vi "Begin.vi"(8 "error in":errorcluster) -> (0 "error out":errorcluster)   [LabVIEW 2018]
doc: "Called before other user functions, this VI is expected to open initial I/O refnums, load in file data, and do all program initialization. Notice that the <B>error out</B> terminal is simply used for data flow. Wiring it to other structures or subVIs ensures that this VI runs first."
uses:
  <vilib>/Rock Robotics/WPI/ThirdParty/Phoenix-LabVIEW/Motor Controller/Controls/CTRE_Phoenix_MotorControl_EnhancedMotorControllerConfigurables.ctl
  <vilib>/Rock Robotics/WPI/ThirdParty/Phoenix-LabVIEW/Motor Controller/Controls/CTRE_Phoenix_MotorControl_BaseConfigurables.ctl
  <vilib>/Rock Robotics/WPI/ThirdParty/Phoenix-LabVIEW/Motor Controller/Controls/CTRE_Phoenix_MotorControl_VelocityMeasurementPeriod.ctl
  <vilib>/Rock Robotics/WPI/ThirdParty/Phoenix-LabVIEW/Motor Controller/Controls/CTRE_Phoenix_MotorControl_SlotStructure.ctl
  <vilib>/Rock Robotics/WPI/ThirdParty/Phoenix-LabVIEW/Motor Controller/Controls/CTRE_Phoenix_MotorControl_FilterStruct.ctl
  <vilib>/Rock Robotics/WPI/ThirdParty/Phoenix-LabVIEW/Motor Controller/Controls/CTRE_Phoenix_MotorControl_RemoteSourceType.ctl
  <vilib>/Rock Robotics/WPI/ThirdParty/Phoenix-LabVIEW/Controls/CTRE_Phoenix_CustomParamConfiguration.ctl
  <vilib>/Rock Robotics/WPI/ThirdParty/Phoenix-LabVIEW/Motor Controller/Controls/CTRE_Phoenix_MotorControl_FeedbackDevice.ctl
  <vilib>/Rock Robotics/WPI/ThirdParty/Phoenix-LabVIEW/Motor Controller/Controls/CTRE_Phoenix_MotorControl_SensorTermFeedbackDevice_Enhanced.ctl
  <vilib>/Rock Robotics/WPI/ThirdParty/Phoenix-LabVIEW/Motor Controller/Controls/CTRE_Phoenix_MotorControl_LimitSwitchNormal.ctl
  <vilib>/Rock Robotics/WPI/ThirdParty/Phoenix-LabVIEW/Motor Controller/Controls/CTRE_Phoenix_MotorControl_LimitSwitchSource_Local.ctl
  <vilib>/Rock Robotics/WPI/ThirdParty/Phoenix-LabVIEW/Motor Controller/Controls/CTRE_Phoenix_MotorControl_MotorControllerConfigurables.ctl
  <vilib>/Rock Robotics/WPI/ThirdParty/Phoenix-LabVIEW/Motor Controller/Controls/CTRE_Phoenix_MotorControl_RemoteFeedbackDevice.ctl
  <vilib>/Rock Robotics/WPI/ThirdParty/Phoenix-LabVIEW/Motor Controller/Controls/CTRE_Phoenix_MotorControl_SensorTermFeedbackDevice.ctl
  <vilib>/Rock Robotics/WPI/ThirdParty/Phoenix-LabVIEW/Motor Controller/Controls/CTRE_Phoenix_MotorControl_LimitSwitchSource.ctl
  <vilib>/Rock Robotics/WPI/DriverStation/WPI_DriverStationRobotMode2.ctl
  <vilib>/Rock Robotics/WPI/Joystick/WPI_JoystickDeviceEnum.ctl
  <vilib>/Rock Robotics/WPI/Solenoid/WPI_SolenoidChannel.ctl
  <vilib>/Rock Robotics/SystemInterfaces/AI/FPGA_AIChannel.ctl
  <vilib>/Rock Robotics/WPI/ThirdParty/Phoenix-LabVIEW/Motor Controller/Controls/CTRE_Phoenix_MotorControl_NeutralMode.ctl
  <vilib>/Rock Robotics/WPI/SafetyOutput/WPI_SafetyOutputConfigMenu.ctl
  Robot Global Data.vi
  RefNums_DriverStation.vi
  <vilib>/Rock Robotics/Network Tables/NT Write String Array.vi
  <vilib>/Rock Robotics/WPI/Solenoid/WPI_SolenoidOpenDouble.vi
  RefNums_Actuators.vi
  <vilib>/Rock Robotics/WPI/Utilities/WPI_GetSetVariantRefNum.vi
  RefNums_Sensors.vi
  <vilib>/Rock Robotics/WPI/Solenoid/WPI_SolenoidOpenSingle.vi
  <vilib>/Rock Robotics/WPI/RobotDrive/WPI_RobotDriveOpen2MotorWithExistingMotors.vi
panel:
  in  "Victor Enhanced Control":T1={"Base Configurables"={"openLoopRamp"=0.0, "closedLoopRamp"=0.0, "peakOutputForward"=1.0, "peakOutputReverse"=-1.0, "nominalOutputForward"=0.0, "nominalOutputReverse"=0.0, "neutralDeadband"=0.04, "voltageCompSaturation"=0.0, "voltageMeasurementFilter"=32, "velocityMeasurementPeriod"=100, "velocityMeasurementWindow"=64, "forwardSoftLimitThreshold"=0, "reverseSoftLimitThreshold"=0, "forwardSoftLimitEnable"=FALSE, "reverseSoftLimitEnable"=FALSE, "slot0"={"P"=0.0, "I"=0.0, "D"=0.0, "F"=0.0, "integralZone"=0.0, "allowableClosedLoopError"=0, "maxIntegralAccumulator"=0.0, "closedLoopPeakOutput"=1.0, "closedLoopPeriod"=1}, "slot1"={"P"=0.0, "I"=0.0, "D"=0.0, "F"=0.0, "integralZone"=0.0, "allowableClosedLoopError"=0, "maxIntegralAccumulator"=0.0, "closedLoopPeakOutput"=1.0, "closedLoopPeriod"=1}, "slot2"={"P"=0.0, "I"=0.0, "D"=0.0, "F"=0.0, "integralZone"=0.0, "allowableClosedLoopError"=0, "maxIntegralAccumulator"=0.0, "closedLoopPeakOutput"=1.0, "closedLoopPeriod"=1}, "slot3"={"P"=0.0, "I"=0.0, "D"=0.0, "F"=0.0, "integralZone"=0.0, "allowableClosedLoopError"=0, "maxIntegralAccumulator"=0.0, "closedLoopPeakOutput"=1.0, "closedLoopPeriod"=1}, "auxPIDPolarity"=FALSE, "remoteFilter0"={"remoteSensorDeviceID"=0, "remoteSensorSource"=enum."Off"}, "remoteFilter1"={"remoteSensorDeviceID"=0, "remoteSensorSource"=enum."Off"}, "motionCruiseVelocity"=0, "motionAcceleration"=0, "motionProfileTrajectoryPeriod"=0, "feedbackNotContinuous"=FALSE, "remoteSensorClosedLoopDisableNeutralOnLOS"=FALSE, "clearPositionOnLimitF"=FALSE, "clearPositionOnLimitR"=FALSE, "clearPositionOnQuadIdx"=FALSE, "limitSwitchDisableNeutralOnLOS"=FALSE, "softLimitDisableNeutralOnLOS"=FALSE, "pulseWidthPeriod_EdgesPerRot"=1, "pulseWidthPeriod_FilterWindowSz"=1, "customParam"={"customParam0"=0, "customParam1"=0}, "trajectoryInterpolationEnable"=TRUE}, "primaryPID"={"selectedFeedbackCoefficient"=1.0, "selectedFeedbackSensor"=11}, "auxiliaryPID"={"selectedFeedbackCoefficient"=1.0, "selectedFeedbackSensor"=11}, "sum 0 term"=11, "sum 1 term"=11, "diff 0 term "=11, "diff 1 term"=11, "forwardLimitSwitchDeviceID"=0, "reverseLimitSwitchDeviceID"=0, "forwardLimitSwitchNormal"=enum."Normally Open", "reverseLimitSwitchNormal"=enum."Normally Open", "forwardLimitSwitchSource"=3, "reverseLimitSwitchSource"=3} {"diff 1 term" items=["Remote Source 0"=11, "Remote Source 1"=12, "Software Emulated"=15]; "diff 0 term" items=["Remote Source 0"=11, "Remote Source 1"=12, "Software Emulated"=15]; "sum 1 term" items=["Remote Source 0"=11, "Remote Source 1"=12, "Software Emulated"=15]; "sum 0 term" items=["Remote Source 0"=11, "Remote Source 1"=12, "Software Emulated"=15]; "reverseLimitSwitchSource" items=["Remote Talon SRX"=1, "Remote CANifier"=2, "Deactivated"=3]; "forwardLimitSwitchSource" items=["Remote Talon SRX"=1, "Remote CANifier"=2, "Deactivated"=3]; "auxiliaryPID"."selectedFeedbackSensor" items=["Sensor Sum (S0 + S1)"=9, "Sensor Difference (D0 - D1)"=10, "Remote Source 0"=11, "Remote Source 1"=12, "Software Emulated"=15]; "primaryPID"."selectedFeedbackSensor" items=["Sensor Sum (S0 + S1)"=9, "Sensor Difference (D0 - D1)"=10, "Remote Source 0"=11, "Remote Source 1"=12, "Software Emulated"=15]; "Base Configurables"."velocityMeasurementPeriod" items=["Period_1ms"=1, "Period_2ms"=2, "Period_5ms"=5, "Period_10ms"=10, "Period_20ms"=20, "Period_25ms"=25, "Period_50ms"=50, "Period_100ms"=100]}
  in  "Talon Enhanced Config":T12={"Base Configurables"={"openLoopRamp"=0.0, "closedLoopRamp"=0.0, "peakOutputForward"=1.0, "peakOutputReverse"=-1.0, "nominalOutputForward"=0.0, "nominalOutputReverse"=0.0, "neutralDeadband"=0.04, "voltageCompSaturation"=0.0, "voltageMeasurementFilter"=32, "velocityMeasurementPeriod"=100, "velocityMeasurementWindow"=64, "forwardSoftLimitThreshold"=0, "reverseSoftLimitThreshold"=0, "forwardSoftLimitEnable"=FALSE, "reverseSoftLimitEnable"=FALSE, "slot0"={"P"=0.0, "I"=0.0, "D"=0.0, "F"=0.0, "integralZone"=0.0, "allowableClosedLoopError"=0, "maxIntegralAccumulator"=0.0, "closedLoopPeakOutput"=1.0, "closedLoopPeriod"=1}, "slot1"={"P"=0.0, "I"=0.0, "D"=0.0, "F"=0.0, "integralZone"=0.0, "allowableClosedLoopError"=0, "maxIntegralAccumulator"=0.0, "closedLoopPeakOutput"=1.0, "closedLoopPeriod"=1}, "slot2"={"P"=0.0, "I"=0.0, "D"=0.0, "F"=0.0, "integralZone"=0.0, "allowableClosedLoopError"=0, "maxIntegralAccumulator"=0.0, "closedLoopPeakOutput"=1.0, "closedLoopPeriod"=1}, "slot3"={"P"=0.0, "I"=0.0, "D"=0.0, "F"=0.0, "integralZone"=0.0, "allowableClosedLoopError"=0, "maxIntegralAccumulator"=0.0, "closedLoopPeakOutput"=1.0, "closedLoopPeriod"=1}, "auxPIDPolarity"=FALSE, "remoteFilter0"={"remoteSensorDeviceID"=0, "remoteSensorSource"=enum."Off"}, "remoteFilter1"={"remoteSensorDeviceID"=0, "remoteSensorSource"=enum."Off"}, "motionCruiseVelocity"=0, "motionAcceleration"=0, "motionProfileTrajectoryPeriod"=0, "feedbackNotContinuous"=FALSE, "remoteSensorClosedLoopDisableNeutralOnLOS"=FALSE, "clearPositionOnLimitF"=FALSE, "clearPositionOnLimitR"=FALSE, "clearPositionOnQuadIdx"=FALSE, "limitSwitchDisableNeutralOnLOS"=FALSE, "softLimitDisableNeutralOnLOS"=FALSE, "pulseWidthPeriod_EdgesPerRot"=1, "pulseWidthPeriod_FilterWindowSz"=1, "customParam"={"customParam0"=0, "customParam1"=0}, "trajectoryInterpolationEnable"=TRUE}, "primaryPID"={"selectedFeedbackCoefficient"=1.0, "selectedFeedbackSensor"=0}, "auxiliaryPID"={"selectedFeedbackCoefficient"=1.0, "selectedFeedbackSensor"=0}, "sum0Term"=0, "sum1Term"=0, "diff0Term"=0, "diff1Term"=0, "forwardLimitSwitchNormal"=enum."Normally Open", "reverseLimitSwitchNormal"=enum."Normally Open", "forwardLimitSwitchDeviceID"=0, "reverseLimitSwitchDeviceID"=0, "forwardLimitSwitchSource"=enum."Feedback Connector", "reverseLimitSwitchSource"=enum."Feedback Connector", "peakCurrentLimit"=1, "peakCurrentDuration"=1, "continuousCurrentLimit"=1} {"diff1Term" items=["QuadEncoder"=0, "Analog"=2, "Tachometer"=4, "Pulse Width Encoded Position"=8, "Remote Source 0"=11, "Remote Source 1"=12, "Software Emulated"=15]; "diff0Term" items=["QuadEncoder"=0, "Analog"=2, "Tachometer"=4, "Pulse Width Encoded Position"=8, "Remote Source 0"=11, "Remote Source 1"=12, "Software Emulated"=15]; "sum1Term" items=["QuadEncoder"=0, "Analog"=2, "Tachometer"=4, "Pulse Width Encoded Position"=8, "Remote Source 0"=11, "Remote Source 1"=12, "Software Emulated"=15]; "sum0Term" items=["QuadEncoder"=0, "Analog"=2, "Tachometer"=4, "Pulse Width Encoded Position"=8, "Remote Source 0"=11, "Remote Source 1"=12, "Software Emulated"=15]; "auxiliaryPID"."selectedFeedbackSensor" items=["QuadEncoder"=0, "Analog"=2, "Tachometer"=4, "Pulse Width Encoded Position"=8, "Sensor Sum (S0 + S1)"=9, "Sensor Difference (D0 - D1)"=10, "Remote Source 0"=11, "Remote Source 1"=12, "Software Emulated"=15]; "primaryPID"."selectedFeedbackSensor" items=["QuadEncoder"=0, "Analog"=2, "Tachometer"=4, "Pulse Width Encoded Position"=8, "Sensor Sum (S0 + S1)"=9, "Sensor Difference (D0 - D1)"=10, "Remote Source 0"=11, "Remote Source 1"=12, "Software Emulated"=15]; "Base Configurables"."velocityMeasurementPeriod" items=["Period_1ms"=1, "Period_2ms"=2, "Period_5ms"=5, "Period_10ms"=10, "Period_20ms"=20, "Period_25ms"=25, "Period_50ms"=50, "Period_100ms"=100]}
  # "Sum and Diff terms are ways to select more than one sensor as a feedback device. \n Sum 0 is the first feedback device to be used for the Sum term, \n Sum 1 is the feedback device to be added to Sum 0 for the Sum term\n Diff 0 and Diff 1 work in a similar manner"
  # "These are only applicable\nif using a remote limit switch.\n\nLocal limit switches/no limit\nswitches do not use this"
  # "False: Primary Output = PID[0] + PID[1]  ---  Auxiliary Output = PID[0] - PID[1]\nTrue:  Primary Output = PID[0] - PID[1] --- Auxiliary Output = PID[0] + PID[1]"
  # "Enable the motion profile executor to perform linear interpolation between profile points.  Defaults to True."
  # "Sum and Diff terms are ways to select more than one sensor as a feedback device. \n Sum 0 is the first feedback device to be used for the Sum term.\n Sum 1 is the feedback device to be added to Sum 0 for the Sum term.\n Diff 0 and Diff 1 work in a similar manner."
  # "These are only applicable\nif using a remote limit switch.\n\nLocal limit switches/no limit\nswitches do not use this."
  # "Current is below Continuous threshold AND\n\n(Requested output is weaker** than applied motor\noutput OR is in the opposite direction).\n/\nMotor output is set to requested output."
  # "Current is above Peak* Threshold for Peak Duration.\n/\nReduce motor output (towards neutral)."
  # "Current is below Continuous threshold.\n/\nRamp motor output towards requested output."
  # "Current is above Continuous threshold.\n/\nReduce motor output (towards neutral)."
  # "Current Limiting is NOT enabled\nby default.\nCall this VI to enable."
  # "*If the configured Peak Threshold is less than the Continuous Threshold, the applied Peak Threshold is set equal to the Configured Continuous Threshold in firmware.\n** Both requested output and applied motor output are in the same direction, and requested output is closer to neutral."
  # "False: Primary Output = PID[0] + PID[1]  ---  Auxiliary Output = PID[0] - PID[1]\nTrue:  Primary Output = PID[0] - PID[1] --- Auxiliary Output = PID[0] + PID[1]"
  # "Enable the motion profile executor to perform linear interpolation between profile points.  Defaults to True."
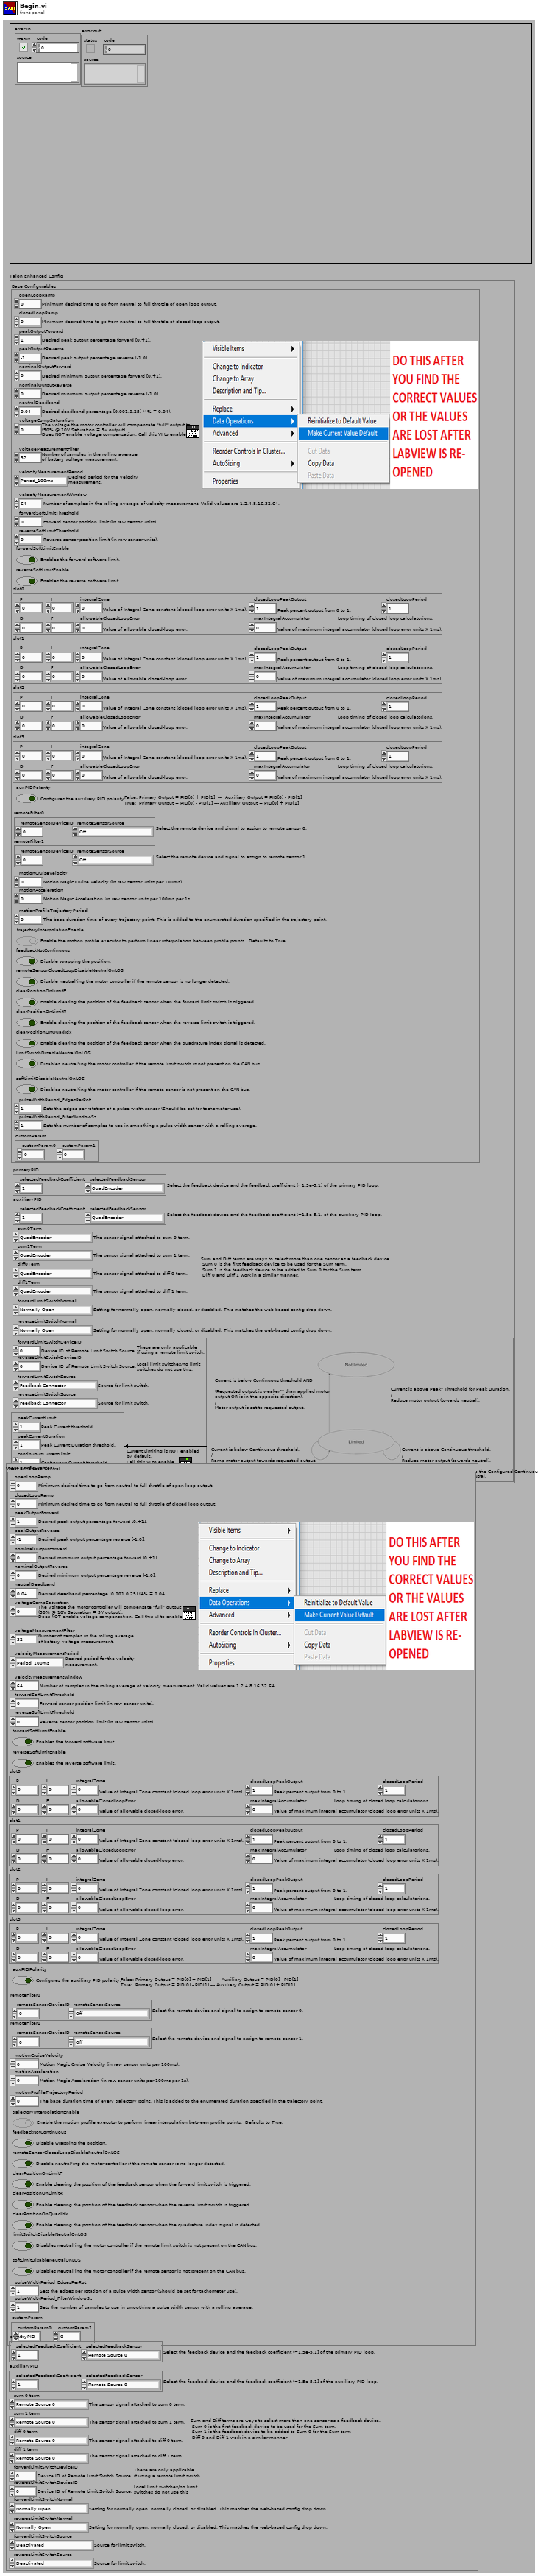
[diagram p1: front panel]
types:
  T1 = typedef "CTRE_Phoenix_MotorControl_MotorControllerConfigurables.ctl" = cluster{"Base Configurables":T2, "primaryPID":cluster{"selectedFeedbackCoefficient":dbl, "selectedFeedbackSensor":T8}, "auxiliaryPID":cluster{"selectedFeedbackCoefficient":dbl, "selectedFeedbackSensor":T8}, "sum 0 term":T9, "sum 1 term":T9, "diff 0 term ":T9, "diff 1 term":T9, "forwardLimitSwitchDeviceID":i32, "reverseLimitSwitchDeviceID":i32, "forwardLimitSwitchNormal":T10, "reverseLimitSwitchNormal":T10, "forwardLimitSwitchSource":T11, "reverseLimitSwitchSource":T11}
  T2 = typedef "CTRE_Phoenix_MotorControl_BaseConfigurables.ctl" = cluster{"openLoopRamp":dbl, "closedLoopRamp":dbl, "peakOutputForward":dbl, "peakOutputReverse":dbl, "nominalOutputForward":dbl, "nominalOutputReverse":dbl, "neutralDeadband":dbl, "voltageCompSaturation":dbl, "voltageMeasurementFilter":i32, "velocityMeasurementPeriod":T3, "velocityMeasurementWindow":i32, "forwardSoftLimitThreshold":i32, "reverseSoftLimitThreshold":i32, "forwardSoftLimitEnable":bool, "reverseSoftLimitEnable":bool, "slot0":T4, "slot1":T4, "slot2":T4, "slot3":T4, "auxPIDPolarity":bool, "remoteFilter0":T5, "remoteFilter1":T5, "motionCruiseVelocity":i32, "motionAcceleration":i32, "motionProfileTrajectoryPeriod":i32, "feedbackNotContinuous":bool, "remoteSensorClosedLoopDisableNeutralOnLOS":bool, "clearPositionOnLimitF":bool, "clearPositionOnLimitR":bool, "clearPositionOnQuadIdx":bool, "limitSwitchDisableNeutralOnLOS":bool, "softLimitDisableNeutralOnLOS":bool, "pulseWidthPeriod_EdgesPerRot":i32, "pulseWidthPeriod_FilterWindowSz":i32, "customParam":T7, "trajectoryInterpolationEnable":bool}
  T3 = typedef "CTRE_Phoenix_MotorControl_VelocityMeasurementPeriod.ctl" = u16
  T4 = typedef "CTRE_Phoenix_MotorControl_SlotStructure.ctl" = cluster{"P":dbl, "I":dbl, "D":dbl, "F":dbl, "integralZone":dbl, "allowableClosedLoopError":i32, "maxIntegralAccumulator":dbl, "closedLoopPeakOutput":dbl, "closedLoopPeriod":i32}
  T5 = typedef "CTRE_Phoenix_MotorControl_FilterStruct.ctl" = cluster{"remoteSensorDeviceID":u8, "remoteSensorSource":T6}
  T6 = typedef "CTRE_Phoenix_MotorControl_RemoteSourceType.ctl" = enum16{"Off", "Talon SRX Selected Sensor", "Pigeon IMU Yaw", "Pigeon IMU Pitch", "Pigeon IMU Roll", "CANifier Quadrature", "CANifier PWM Input 0", "CANifier PWM Input 1", "CANifier PWM Input 2", "CANifier PWM Input 3", "Gadgeteer Pigeon Yaw", "Gadgeteer Pigeon Pitch", "Gadgeteer Pigeon Roll"}
  T7 = typedef "CTRE_Phoenix_CustomParamConfiguration.ctl" = cluster{"customParam0":i32, "customParam1":i32}
  T8 = typedef "CTRE_Phoenix_MotorControl_RemoteFeedbackDevice.ctl" = i8
  T9 = typedef "CTRE_Phoenix_MotorControl_SensorTermFeedbackDevice.ctl" = i8
  T10 = typedef "CTRE_Phoenix_MotorControl_LimitSwitchNormal.ctl" = enum16{"Normally Open", "Normally Closed", "Disabled"}
  T11 = typedef "CTRE_Phoenix_MotorControl_LimitSwitchSource.ctl" = u16
  T12 = typedef "CTRE_Phoenix_MotorControl_EnhancedMotorControllerConfigurables.ctl" = cluster{"Base Configurables":T2, "primaryPID":cluster{"selectedFeedbackCoefficient":dbl, "selectedFeedbackSensor":T13}, "auxiliaryPID":cluster{"selectedFeedbackCoefficient":dbl, "selectedFeedbackSensor":T13}, "sum0Term":T14, "sum1Term":T14, "diff0Term":T14, "diff1Term":T14, "forwardLimitSwitchNormal":T10, "reverseLimitSwitchNormal":T10, "forwardLimitSwitchDeviceID":i32, "reverseLimitSwitchDeviceID":i32, "forwardLimitSwitchSource":T15, "reverseLimitSwitchSource":T15, "peakCurrentLimit":i32, "peakCurrentDuration":i32, "continuousCurrentLimit":i32}
  T13 = typedef "CTRE_Phoenix_MotorControl_FeedbackDevice.ctl" = i8
  T14 = typedef "CTRE_Phoenix_MotorControl_SensorTermFeedbackDevice_Enhanced.ctl" = i8
  T15 = typedef "CTRE_Phoenix_MotorControl_LimitSwitchSource_Local.ctl" = enum16{"Feedback Connector", "Remote Talon SRX", "Remote CANifier", "Deactivated"}
  T16 = typedef "WPI_SafetyOutputConfigMenu.ctl" = enum16{"Enable", "Disable"}
  T17 = typedef "WPI_JoystickDeviceEnum.ctl" = enum16{"USB 0", "USB 1", "USB 2", "USB 3", "USB 4", "USB 5"}
  T18 = typedef "CTRE_Phoenix_MotorControl_NeutralMode.ctl" = enum8{"EEPROMSetting", "Override to Coast", "Override to Brake"}
  T19 = typedef "FPGA_AIChannel.ctl" = enum8{"AI 0", "AI 1", "AI 2", "AI 3", "AI MXP 0", "AI MXP 1", "AI MXP 2", "AI MXP 3", "Invalid"}
  T20 = typedef "WPI_SolenoidChannel.ctl" = enum8{"Solenoid 0", "Solenoid 1", "Solenoid 2", "Solenoid 3", "Solenoid 4", "Solenoid 5", "Solenoid 6", "Solenoid 7", "Invalid"}
  T21 = typedef "WPI_DriverStationRobotMode2.ctl" = enum16{"Autonomous Disabled", "Autonomous Enabled", "Teleop Disabled", "Teleop Enabled", "Disconnected", "Finish", "Test Disabled", "Test Enabled", "Emergency Stopped"}
  T22 = typedef "WPI_JoystickDevRef.ctl" = cluster{"Device":T17}
  T23 = typedef "WPI_MotorControlDeviceRef.ctl" = cluster{"DeviceStatus":errorcluster, "Type":T24, "PWM":cluster{"PWM Channel":T25, "DeadBand":T26}, "CAN":cluster{"Device Number":u8, "SetOutput VI Ref":variant, "GetOutput VI Ref":variant, "Enable VI Ref":variant, "Disable VI Ref":variant, "Data":variant}, "Invert":bool, "DIO PWM":cluster{"PWM \"Enable\" Channel":T25, "DIOChannel":T27, "PWM Rate":dbl}}
  T24 = typedef "WPI_MotorControlType.ctl" = enum16{"PWM", "CAN", "DIO PWM"}
  T25 = typedef "FPGA_DIOPWMChannel.ctl" = enum8{"PWM 0", "PWM 1", "PWM 2", "PWM 3", "PWM 4", "PWM 5", "PWM 6", "PWM 7", "PWM 8", "PWM 9", "PWM MXP 0", "PWM MXP 1", "PWM MXP 2", "PWM MXP 3", "PWM MXP 4", "PWM MXP 5", "PWM MXP 6", "PWM MXP 7", "PWM MXP 8", "PWM MXP 9", "Invalid"}
  T26 = typedef "WPI_PWMDeadband.ctl" = cluster{"Name":string, "maxPositivePwm":i32, "minPositivePwm":i32, "centerPwm":i32, "maxNegativePwm":i32, "minNegativePwm":i32, "angularRange":u16}
  T27 = typedef "FPGA_DIOChannel.ctl" = enum8{"DIO 0", "DIO 1", "DIO 2", "DIO 3", "DIO 4", "DIO 5", "DIO 6", "DIO 7", "DIO 8", "DIO 9", "DIO MXP 0", "DIO MXP 1", "DIO MXP 2", "DIO MXP 3", "DIO MXP 4", "DIO MXP 5", "DIO MXP 6", "DIO MXP 7", "DIO MXP 8", "DIO MXP 9", "DIO MXP 10", "DIO MXP 11", "DIO MXP 12", "DIO MXP 13", "DIO MXP 14", "DIO MXP 15", "SPI Port CS1", "SPI Port CS2", "SPI Port CS3", "SPI Port MISO", "SPI Port MOSI", "Invalid"}
  T28 = typedef "WPI_RobotDriveDevRef.ctl" = cluster{"DevStatus":errorcluster, "Motors[]":T23[], "Square Inputs":bool, "Max Output":dbl}
  T29 = typedef "WPI_SolenoidDevRef.ctl" = cluster{"DevStatus":errorcluster, "Pneumatics Control Module":u8, "Forward Solenoid Channel":T20, "Reverse Solenoid Channel":T20}
  T30 = typedef "WPI_CompressorDevRef.ctl" = cluster{"DevStatus":errorcluster, "Pneumatics Control Module":u8}
  T31 = typedef "WPI_AnalogChannelDevRef.ctl" = cluster{"DevStatus":errorcluster, "Analog Channel":T19}
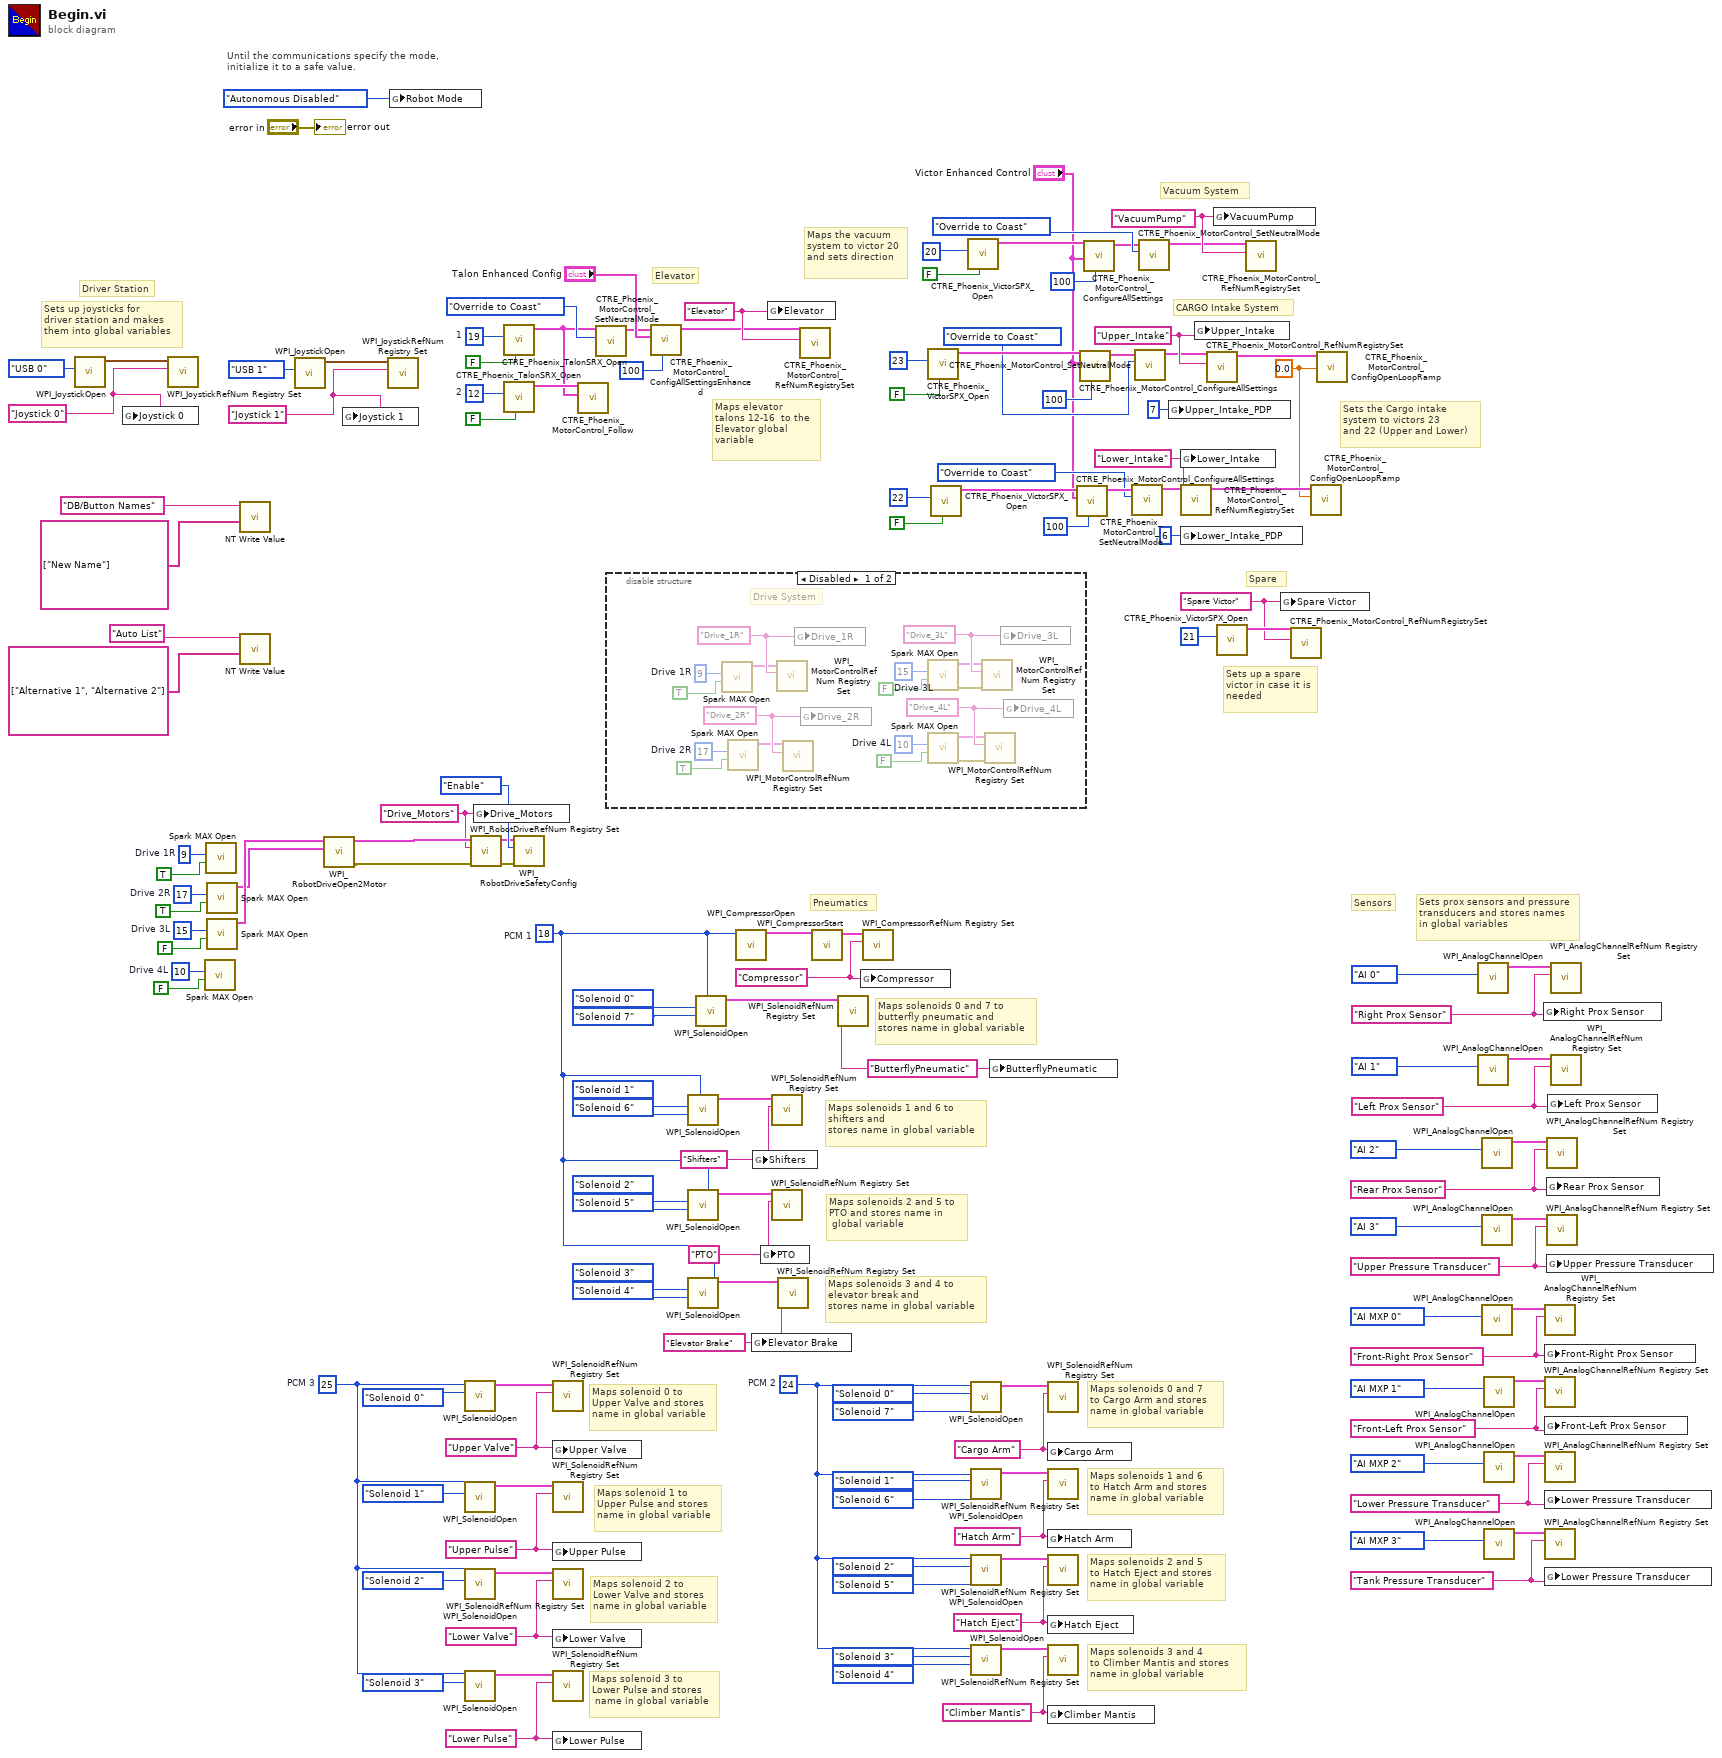
[diagram p0: block diagram]
diagram:
  w5 = "Drive_Motors" ("refnum name")
  w13 = u8 10  # Drive 4L
  w14 = u8 15  # Drive 3L
  w16 = u8 17  # Drive 2R
  w18 = u8 9  # Drive 1R
  w20 = "Joystick 1" ("refnum name")
  w39 = u8 12  # 2
  w44 = "Tank Pressure Transducer" ("refnum name")
  w47 = "Lower Pressure Transducer" ("refnum name")
  w50 = "Front-Left Prox Sensor" ("refnum name")
  w53 = "Front-Right Prox Sensor" ("refnum name")
  w57 = "Lower Pulse" ("ButterflyPneumatic")
  w60 = "Lower Valve" ("ButterflyPneumatic")
  w63 = "Upper Valve" ("ButterflyPneumatic")
  w67 = "Climber Mantis" ("ButterflyPneumatic")
  w71 = "Hatch Eject" ("ButterflyPneumatic")
  w75 = "Hatch Arm" ("ButterflyPneumatic")
  w56 = u8 25  # PCM 3
  w66 = u8 24  # PCM 2
  w80 = "Elevator Brake" ("ButterflyPneumatic")
  w84 = "PTO" ("ButterflyPneumatic")
  w88 = "Spare Victor" ("refnum name")
  w91 = "Upper Pressure Transducer" ("refnum name")
  w94 = "Rear Prox Sensor" ("refnum name")
  w97 = "Left Prox Sensor" ("refnum name")
  w100 = "Right Prox Sensor" ("refnum name")
  w103 = "Elevator" ("refnum name")
  w105 = u8 19  # 1
  w108 = 0.0 ("secondsFromNeutralToFull")
  w111 = "Lower_Intake" ("refnum name")
  w112 = "Upper_Intake" ("refnum name")
  w117 = "Cargo Arm" ("ButterflyPneumatic")
  w121 = "VacuumPump" ("refnum name")
  w124 = "Upper Pulse" ("ButterflyPneumatic")
  w127 = "Shifters" ("ButterflyPneumatic")
  w131 = "Compressor" ("Compressor")
  w132 = "ButterflyPneumatic" ("ButterflyPneumatic")
  w79 = u8 18  # PCM 1
  w138 = "Joystick 0" ("refnum name")
  # "Sets the Cargo intake \nsystem to victors 23 \nand 22 (Upper and Lower)"
  # "Maps the vacuum\nsystem to victor 20\nand sets direction"
  # "Sets up a spare\nvictor in case it is\nneeded"
  # "Sets up joysticks for\ndriver station and makes\nthem into global variables"
  # "Maps elevator\ntalons 12-16  to the \nElevator global\nvariable"
  # "Maps solenoids 3 and 4\nto Climber Mantis and stores \nname in global variable"
  # "Maps solenoids 2 and 5\nto Hatch Eject and stores \nname in global variable"
  # "Maps solenoids 1 and 6\nto Hatch Arm and stores \nname in global variable"
  # "Maps solenoids 0 and 7\nto Cargo Arm and stores \nname in global variable"
  # "Maps solenoid 0 to\nUpper Valve and stores \nname in global variable"
  # "Maps solenoid 1 to\nUpper Pulse and stores \nname in global variable"
  # "Maps solenoid 2 to\nLower Valve and stores \nname in global variable"
  # "Maps solenoid 3 to\nLower Pulse and stores\n name in global variable"
  # "Maps solenoids 3 and 4 to\nelevator break and \nstores name in global variable"
  # "Maps solenoids 2 and 5 to\nPTO and stores name in\n global variable"
  # "Maps solenoids 1 and 6 to\nshifters and \nstores name in global variable"
  # "Maps solenoids 0 and 7 to\nbutterfly pneumatic and \nstores name in global variable"
  # "Sets prox sensors and pressure\ntransducers and stores names \nin global variables"
  # "Spare"
  # "CARGO Intake System"
  # "Vacuum System"
  # "Elevator"
  # "Sensors"
  # "Pneumatics"
  # "Driver Station"
  # "Until the communications specify the mode,\ninitialize it to a safe value."
  n1 = call <vilib>:"WPI_JoystickOpen.vi"("JoystickDevice"=WPI_JoystickDeviceEnum."USB 0") -> ("JoystickDevRef"=w145:T22)  [unwired: 10 in]
  n2 = global write "RefNums_DriverStation.vi" "Joystick 0"(w138) -> ()
  n3 = call <vilib>:"WPI_JoystickRefNum Registry Set.vi"("refnum name"=w138, "JoystickDevRef"=w145) -> ()  [unwired: 8 in, 2 out]
  n4 = call <vilib>:"Spark MAX Open.vi"("Invert"=FALSE, "Device Number"=w13) -> ()  [unwired: 8 in, 2 out]
  n5 = call <vilib>:"Spark MAX Open.vi"("Invert"=TRUE, "Device Number"=w18) -> ()  [unwired: 8 in, 2 out]
  n6 = call <vilib>:"Spark MAX Open.vi"("Invert"=TRUE, "Device Number"=w16) -> ("MotorControlDeviceRef"=w3:T23)  [unwired: 8 in, 1 out]
  n7 = call <vilib>:"Spark MAX Open.vi"("Invert"=FALSE, "Device Number"=w14) -> ("MotorControlDeviceRef"=w4:T23)  [unwired: 8 in, 1 out]
  n8 = call-poly <vilib>:"NT Write Value.vi"("String Array"=string[] ["New Name"], "Name"="DB/Button Names") -> ()  [unwired: 9 in, 1 out]
  n9 = call-poly <vilib>:"NT Write Value.vi"("String Array"=string[] ["Alternative 1", "Alternative 2"], "Name"="Auto List") -> ()  [unwired: 9 in, 1 out]
  n10 = call <vilib>:"WPI_JoystickOpen.vi"("JoystickDevice"=WPI_JoystickDeviceEnum."USB 1") -> ("JoystickDevRef"=w19:T22)  [unwired: 10 in]
  n11 = call-poly <vilib>:"WPI_RobotDriveOpen2Motor.vi"("Right Motor Dev Ref"=w3, "Left Motor Dev Ref"=w4) -> ("error out"=w6:errorcluster, "RobotDriveDevRef"=w7:T28)  [unwired: 8 in]
  n12 = global write "RefNums_DriverStation.vi" "Joystick 1"(w20) -> ()
  n13 = call <vilib>:"WPI_JoystickRefNum Registry Set.vi"("refnum name"=w20, "JoystickDevRef"=w19) -> ()  [unwired: 8 in, 2 out]
  n14 = global write "Robot Global Data.vi" "Robot Mode"(WPI_DriverStationRobotMode2."Autonomous Disabled" ("Robot Mode")) -> ()
  n15 = call-poly <vilib>:"WPI_SolenoidOpen.vi"("Solenoid Channel"=WPI_SolenoidChannel."Solenoid 0" ("Forward Solenoid Channel"), "Pneumatics Control Module (0)"=w56) -> ("SolenoidDevRef"=w64:T29)  [unwired: 8 in, 1 out]
  n16 = call-poly <vilib>:"WPI_SolenoidOpen.vi"("Solenoid Channel"=WPI_SolenoidChannel."Solenoid 1" ("Forward Solenoid Channel"), "Pneumatics Control Module (0)"=w56) -> ("SolenoidDevRef"=w125:T29)  [unwired: 8 in, 1 out]
  n17 = call-poly <vilib>:"WPI_SolenoidOpen.vi"("Solenoid Channel"=WPI_SolenoidChannel."Solenoid 2" ("Forward Solenoid Channel"), "Pneumatics Control Module (0)"=w56) -> ("SolenoidDevRef"=w61:T29)  [unwired: 8 in, 1 out]
  n18 = call-poly <vilib>:"WPI_SolenoidOpen.vi"("Solenoid Channel"=WPI_SolenoidChannel."Solenoid 3" ("Forward Solenoid Channel"), "Pneumatics Control Module (0)"=w56) -> ("SolenoidDevRef"=w58:T29)  [unwired: 8 in, 1 out]
  n19 = call <vilib>:"WPI_RobotDriveRefNum Registry Set.vi"("error in (no error)"=w6, "refnum name"=w5, "RobotDriveDevRef"=w7) -> ("error out"=w8:errorcluster, "RobotDriveDevRef"=w9:T28)  [unwired: 7 in]
  n20 = global write "RefNums_Actuators.vi" "Drive_Motors"(w5) -> ()
  n21 = call <vilib>:"CTRE_Phoenix_TalonSRX_Open.vi"("Invert"=FALSE, "Device Number"=w105) -> ("CAN Talon SRX Ref"=w1:T23)  [unwired: 8 in, 1 out]
  n22 = call <vilib>:"CTRE_Phoenix_TalonSRX_Open.vi"("Invert"=FALSE, "Device Number"=w39) -> ("CAN Talon SRX Ref"=w2:T23)  [unwired: 8 in, 1 out]
  n23 = call <vilib>:"WPI_RobotDriveSafetyConfig.vi"("error in (no error)"=w8, "mode"=WPI_SafetyOutputConfigMenu."Enable", "RobotDriveDevRef"=w9) -> ()  [unwired: 7 in, 2 out]
  n24 = call <vilib>:"WPI_SolenoidRefNum Registry Set.vi"("refnum name"=w63, "SolenoidDevRef"=w64) -> ()  [unwired: 8 in, 2 out]
  n25 = global write "RefNums_Actuators.vi" "Upper Valve"(w63) -> ()
  n26 = call <vilib>:"WPI_SolenoidRefNum Registry Set.vi"("refnum name"=w124, "SolenoidDevRef"=w125) -> ()  [unwired: 8 in, 2 out]
  n27 = global write "RefNums_Actuators.vi" "Upper Pulse"(w124) -> ()
  n28 = call <vilib>:"WPI_SolenoidRefNum Registry Set.vi"("refnum name"=w60, "SolenoidDevRef"=w61) -> ()  [unwired: 8 in, 2 out]
  n29 = global write "RefNums_Actuators.vi" "Lower Valve"(w60) -> ()
  n30 = call <vilib>:"WPI_SolenoidRefNum Registry Set.vi"("refnum name"=w57, "SolenoidDevRef"=w58) -> ()  [unwired: 8 in, 2 out]
  n31 = global write "RefNums_Actuators.vi" "Lower Pulse"(w57) -> ()
  n32 = call <vilib>:"CTRE_Phoenix_MotorControl_Follow.vi"("Master Controller to Follow"=w1, "PhoenixMotorControlDevRef"=w2) -> ()  [unwired: 8 in, 2 out]
  n33 = call <vilib>:"CTRE_Phoenix_MotorControl_SetNeutralMode.vi"("Motor Control Neutral Mode"=CTRE_Phoenix_MotorControl_NeutralMode."Override to Coast", "PhoenixMotorControlDevRef"=w1) -> ("PhoenixMotorControlDevRef"=w42:T23)  [unwired: 8 in, 1 out]
  n34 = disable-structure shown="Disabled" {
    frame Disabled {
      w152 = "Drive_4L" ("refnum name")
      w155 = "Drive_3L" ("refnum name")
      w156 = "Drive_2R" ("refnum name")
      w159 = u8 10  # Drive 4L
      w160 = u8 15  # Drive 3L
      w164 = u8 17  # Drive 2R
      w161 = "Drive_1R" ("refnum name")
      w165 = u8 9  # Drive 1R
      # "Drive System"
      n35 = call <vilib>:"Spark MAX Open.vi"("Invert"=TRUE, "Device Number"=w165) -> ("MotorControlDeviceRef"=w154:T23)  [unwired: 8 in, 1 out]
      n36 = call <vilib>:"Spark MAX Open.vi"("Invert"=TRUE, "Device Number"=w164) -> ("MotorControlDeviceRef"=w153:T23)  [unwired: 8 in, 1 out]
      n37 = call <vilib>:"WPI_MotorControlRefNum Registry Set.vi"("refnum name"=w161, "MotorControlDevRef"=w154) -> ()  [unwired: 8 in, 2 out]
      n38 = call <vilib>:"WPI_MotorControlRefNum Registry Set.vi"("refnum name"=w156, "MotorControlDevRef"=w153) -> ()  [unwired: 8 in, 2 out]
      n39 = global write "RefNums_Actuators.vi" "Drive_1R"(w161) -> ()
      n40 = global write "RefNums_Actuators.vi" "Drive_2R"(w156) -> ()
      n41 = call <vilib>:"Spark MAX Open.vi"("Invert"=FALSE, "Device Number"=w160) -> ("error out"=w150:errorcluster, "MotorControlDeviceRef"=w151:T23)  [unwired: 8 in]
      n42 = call <vilib>:"Spark MAX Open.vi"("Invert"=FALSE, "Device Number"=w159) -> ("error out"=w148:errorcluster, "MotorControlDeviceRef"=w149:T23)  [unwired: 8 in]
      n43 = call <vilib>:"WPI_MotorControlRefNum Registry Set.vi"("error in (no error)"=w150, "refnum name"=w155, "MotorControlDevRef"=w151) -> ()  [unwired: 7 in, 2 out]
      n44 = call <vilib>:"WPI_MotorControlRefNum Registry Set.vi"("error in (no error)"=w148, "refnum name"=w152, "MotorControlDevRef"=w149) -> ()  [unwired: 7 in, 2 out]
      n45 = global write "RefNums_Actuators.vi" "Drive_3L"(w155) -> ()
      n46 = global write "RefNums_Actuators.vi" "Drive_4L"(w152) -> ()
    }
    frame Enabled {
    }
  }
  n47 = call <vilib>:"CTRE_Phoenix_MotorControl_ConfigAllSettingsEnhanced.vi"("timeoutMs"=100, "Enhanced Motor Controller Configurables"="Talon Enhanced Config", "PhoenixMotorControlDevRef"=w42) -> ("PhoenixMotorControlDevRef"=w41:T23)  [unwired: 7 in, 1 out]
  n48 = call-poly <vilib>:"WPI_SolenoidOpen.vi"("Reverse Solenoid Channel"=WPI_SolenoidChannel."Solenoid 6", "Forward Solenoid Channel"=WPI_SolenoidChannel."Solenoid 1", "Pneumatics Control Module (0)"=w79) -> ("SolenoidDevRef"=w128:T29)  [unwired: 7 in, 1 out]
  n49 = call-poly <vilib>:"WPI_SolenoidOpen.vi"("Reverse Solenoid Channel"=WPI_SolenoidChannel."Solenoid 5", "Forward Solenoid Channel"=WPI_SolenoidChannel."Solenoid 2", "Pneumatics Control Module (0)"=w79) -> ("SolenoidDevRef"=w85:T29)  [unwired: 7 in, 1 out]
  n50 = call-poly <vilib>:"WPI_SolenoidOpen.vi"("Reverse Solenoid Channel"=WPI_SolenoidChannel."Solenoid 4", "Forward Solenoid Channel"=WPI_SolenoidChannel."Solenoid 3", "Pneumatics Control Module (0)"=w79) -> ("SolenoidDevRef"=w81:T29)  [unwired: 7 in, 1 out]
  n51 = call-poly <vilib>:"WPI_SolenoidOpen.vi"("Reverse Solenoid Channel"=WPI_SolenoidChannel."Solenoid 7", "Forward Solenoid Channel"=WPI_SolenoidChannel."Solenoid 0", "Pneumatics Control Module (0)"=w79) -> ("SolenoidDevRef"=w134:T29)  [unwired: 7 in, 1 out]
  n52 = call <vilib>:"WPI_CompressorOpen.vi"("Pneumatics Control Module (0)"=w79) -> ("CompressorDevRef"=w137:T30)  [unwired: 13 in, 1 out]
  n53 = global write "RefNums_Actuators.vi" "Elevator Brake"(w80) -> ()
  n54 = global write "RefNums_Actuators.vi" "Shifters"(w127) -> ()
  n55 = global write "RefNums_Actuators.vi" "PTO"(w84) -> ()
  n56 = global write "RefNums_Actuators.vi" "Elevator"(w103) -> ()
  n57 = call <vilib>:"WPI_SolenoidRefNum Registry Set.vi"("refnum name"=w127, "SolenoidDevRef"=w128) -> ()  [unwired: 8 in, 2 out]
  n58 = call <vilib>:"WPI_SolenoidRefNum Registry Set.vi"("refnum name"=w84, "SolenoidDevRef"=w85) -> ()  [unwired: 8 in, 2 out]
  n59 = call <vilib>:"WPI_SolenoidRefNum Registry Set.vi"("refnum name"=w80, "SolenoidDevRef"=w81) -> ()  [unwired: 8 in, 2 out]
  n60 = call <vilib>:"CTRE_Phoenix_MotorControl_RefNumRegistrySet.vi"("refnum name"=w103, "PhoenixMotorControlDevRef"=w41) -> ()  [unwired: 8 in, 2 out]
  n61 = call <vilib>:"WPI_CompressorStart.vi"("CompressorDevRef"=w137) -> ("CompressorDevRef"=w133:T30)  [unwired: 9 in, 1 out]
  n62 = call <vilib>:"WPI_SolenoidRefNum Registry Set.vi"("refnum name"=w132, "SolenoidDevRef"=w134) -> ()  [unwired: 8 in, 2 out]
  n63 = global write "RefNums_Actuators.vi" "Compressor"(w131) -> ()
  n64 = call <vilib>:"WPI_CompressorRefNum Registry Set.vi"("refnum name"=w131, "CompressorDevRef"=w133) -> ()  [unwired: 8 in, 2 out]
  n65 = call <vilib>:"CTRE_Phoenix_VictorSPX_Open.vi"("Invert"=FALSE, "Device Number"=u8 23) -> ("CAN Talon SRX Ref"=w27:T23)  [unwired: 8 in, 1 out]
  n66 = call <vilib>:"CTRE_Phoenix_VictorSPX_Open.vi"("Invert"=FALSE, "Device Number"=u8 22) -> ("CAN Talon SRX Ref"=w26:T23)  [unwired: 8 in, 1 out]
  n67 = call <vilib>:"CTRE_Phoenix_VictorSPX_Open.vi"("Invert"=FALSE, "Device Number"=u8 20) -> ("CAN Talon SRX Ref"=w34:T23)  [unwired: 8 in, 1 out]
  n68 = call-poly <vilib>:"WPI_SolenoidOpen.vi"("Reverse Solenoid Channel"=WPI_SolenoidChannel."Solenoid 7", "Forward Solenoid Channel"=WPI_SolenoidChannel."Solenoid 0", "Pneumatics Control Module (0)"=w66) -> ("SolenoidDevRef"=w118:T29)  [unwired: 7 in, 1 out]
  n69 = call-poly <vilib>:"WPI_SolenoidOpen.vi"("Reverse Solenoid Channel"=WPI_SolenoidChannel."Solenoid 6", "Forward Solenoid Channel"=WPI_SolenoidChannel."Solenoid 1", "Pneumatics Control Module (0)"=w66) -> ("SolenoidDevRef"=w76:T29)  [unwired: 7 in, 1 out]
  n70 = call-poly <vilib>:"WPI_SolenoidOpen.vi"("Reverse Solenoid Channel"=WPI_SolenoidChannel."Solenoid 5", "Forward Solenoid Channel"=WPI_SolenoidChannel."Solenoid 2", "Pneumatics Control Module (0)"=w66) -> ("SolenoidDevRef"=w72:T29)  [unwired: 7 in, 1 out]
  n71 = call-poly <vilib>:"WPI_SolenoidOpen.vi"("Reverse Solenoid Channel"=WPI_SolenoidChannel."Solenoid 4", "Forward Solenoid Channel"=WPI_SolenoidChannel."Solenoid 3", "Pneumatics Control Module (0)"=w66) -> ("SolenoidDevRef"=w68:T29)  [unwired: 7 in, 1 out]
  n72 = global write "RefNums_Actuators.vi" "ButterflyPneumatic"(w132) -> ()
  n73 = call <vilib>:"WPI_SolenoidRefNum Registry Set.vi"("refnum name"=w117, "SolenoidDevRef"=w118) -> ()  [unwired: 8 in, 2 out]
  n74 = global write "RefNums_Actuators.vi" "Cargo Arm"(w117) -> ()
  n75 = call <vilib>:"WPI_SolenoidRefNum Registry Set.vi"("refnum name"=w75, "SolenoidDevRef"=w76) -> ()  [unwired: 8 in, 2 out]
  n76 = global write "RefNums_Actuators.vi" "Hatch Arm"(w75) -> ()
  n77 = call <vilib>:"WPI_SolenoidRefNum Registry Set.vi"("refnum name"=w71, "SolenoidDevRef"=w72) -> ()  [unwired: 8 in, 2 out]
  n78 = global write "RefNums_Actuators.vi" "Hatch Eject"(w71) -> ()
  n79 = call <vilib>:"WPI_SolenoidRefNum Registry Set.vi"("refnum name"=w67, "SolenoidDevRef"=w68) -> ()  [unwired: 8 in, 2 out]
  n80 = global write "RefNums_Actuators.vi" "Climber Mantis"(w67) -> ()
  n81 = call <vilib>:"CTRE_Phoenix_MotorControl_ConfigureAllSettings.vi"("timeoutMs"=100, "Motor Controller Configurables"="Victor Enhanced Control", "PhoenixMotorControlDevRef"=w26) -> ("PhoenixMotorControlDevRef"=w29:T23)  [unwired: 7 in, 1 out]
  n82 = call <vilib>:"CTRE_Phoenix_MotorControl_ConfigureAllSettings.vi"("timeoutMs"=100, "Motor Controller Configurables"="Victor Enhanced Control", "PhoenixMotorControlDevRef"=w27) -> ("PhoenixMotorControlDevRef"=w28:T23)  [unwired: 7 in, 1 out]
  n83 = call <vilib>:"CTRE_Phoenix_MotorControl_ConfigureAllSettings.vi"("timeoutMs"=100, "Motor Controller Configurables"="Victor Enhanced Control", "PhoenixMotorControlDevRef"=w34) -> ("PhoenixMotorControlDevRef"=w35:T23)  [unwired: 7 in, 1 out]
  n84 = call <vilib>:"CTRE_Phoenix_MotorControl_SetNeutralMode.vi"("Motor Control Neutral Mode"=CTRE_Phoenix_MotorControl_NeutralMode."Override to Coast", "PhoenixMotorControlDevRef"=w29) -> ("PhoenixMotorControlDevRef"=w30:T23)  [unwired: 8 in, 1 out]
  n85 = call <vilib>:"CTRE_Phoenix_MotorControl_SetNeutralMode.vi"("Motor Control Neutral Mode"=CTRE_Phoenix_MotorControl_NeutralMode."Override to Coast", "PhoenixMotorControlDevRef"=w28) -> ("PhoenixMotorControlDevRef"=w23:T23)  [unwired: 8 in, 1 out]
  n86 = call <vilib>:"CTRE_Phoenix_MotorControl_SetNeutralMode.vi"("Motor Control Neutral Mode"=CTRE_Phoenix_MotorControl_NeutralMode."Override to Coast", "PhoenixMotorControlDevRef"=w35) -> ("PhoenixMotorControlDevRef"=w37:T23)  [unwired: 8 in, 1 out]
  n87 = global write "RefNums_Actuators.vi" "Upper_Intake_PDP"(7 ("Upper_Intake_PDP")) -> ()
  n88 = global write "RefNums_Actuators.vi" "Lower_Intake"(w111) -> ()
  n89 = call <vilib>:"CTRE_Phoenix_MotorControl_RefNumRegistrySet.vi"("refnum name"=w111, "PhoenixMotorControlDevRef"=w30) -> ("PhoenixMotorControlDevRef"=w110:T23)  [unwired: 8 in, 1 out]
  n90 = global write "RefNums_Actuators.vi" "Lower_Intake_PDP"(6 ("Lower_Intake_PDP")) -> ()
  n91 = global write "RefNums_Actuators.vi" "Upper_Intake"(w112) -> ()
  n92 = call <vilib>:"CTRE_Phoenix_MotorControl_RefNumRegistrySet.vi"("refnum name"=w112, "PhoenixMotorControlDevRef"=w23) -> ("PhoenixMotorControlDevRef"=w109:T23)  [unwired: 8 in, 1 out]
  n93 = global write "RefNums_Actuators.vi" "VacuumPump"(w121) -> ()
  n94 = call <vilib>:"CTRE_Phoenix_VictorSPX_Open.vi"("Device Number"=u8 21) -> ("CAN Talon SRX Ref"=w89:T23)  [unwired: 9 in, 1 out]
  n95 = call <vilib>:"CTRE_Phoenix_MotorControl_RefNumRegistrySet.vi"("refnum name"=w121, "PhoenixMotorControlDevRef"=w37) -> ()  [unwired: 8 in, 2 out]
  n96 = global write "RefNums_Actuators.vi" "Spare Victor"(w88) -> ()
  n97 = call <vilib>:"CTRE_Phoenix_MotorControl_RefNumRegistrySet.vi"("refnum name"=w88, "PhoenixMotorControlDevRef"=w89) -> ()  [unwired: 8 in, 2 out]
  n98 = call <vilib>:"CTRE_Phoenix_MotorControl_ConfigOpenLoopRamp.vi"("secondsFromNeutralToFull"=w108, "PhoenixMotorControlDevRef"=w110) -> ()  [unwired: 8 in, 2 out]
  n99 = call <vilib>:"CTRE_Phoenix_MotorControl_ConfigOpenLoopRamp.vi"("secondsFromNeutralToFull"=w108, "PhoenixMotorControlDevRef"=w109) -> ()  [unwired: 8 in, 2 out]
  n100 = call <vilib>:"WPI_AnalogChannelOpen.vi"("Analog Channel"=FPGA_AIChannel."AI 0") -> ("AIDeviceRef"=w102:T31)  [unwired: 9 in, 1 out]
  n101 = call <vilib>:"WPI_AnalogChannelOpen.vi"("Analog Channel"=FPGA_AIChannel."AI 1") -> ("AIDeviceRef"=w99:T31)  [unwired: 9 in, 1 out]
  n102 = call <vilib>:"WPI_AnalogChannelOpen.vi"("Analog Channel"=FPGA_AIChannel."AI 2") -> ("AIDeviceRef"=w96:T31)  [unwired: 9 in, 1 out]
  n103 = call <vilib>:"WPI_AnalogChannelOpen.vi"("Analog Channel"=FPGA_AIChannel."AI 3") -> ("AIDeviceRef"=w93:T31)  [unwired: 9 in, 1 out]
  n104 = call <vilib>:"WPI_AnalogChannelOpen.vi"("Analog Channel"=FPGA_AIChannel."AI MXP 0") -> ("AIDeviceRef"=w55:T31)  [unwired: 9 in, 1 out]
  n105 = call <vilib>:"WPI_AnalogChannelOpen.vi"("Analog Channel"=FPGA_AIChannel."AI MXP 1") -> ("AIDeviceRef"=w52:T31)  [unwired: 9 in, 1 out]
  n106 = call <vilib>:"WPI_AnalogChannelOpen.vi"("Analog Channel"=FPGA_AIChannel."AI MXP 2") -> ("AIDeviceRef"=w49:T31)  [unwired: 9 in, 1 out]
  n107 = call <vilib>:"WPI_AnalogChannelOpen.vi"("Analog Channel"=FPGA_AIChannel."AI MXP 3") -> ("AIDeviceRef"=w46:T31)  [unwired: 9 in, 1 out]
  n108 = global write "RefNums_Sensors.vi" "Right Prox Sensor"(w100) -> ()
  n109 = call <vilib>:"WPI_AnalogChannelRefNum Registry Set.vi"("refnum name"=w53, "AIDeviceRef"=w55) -> ()  [unwired: 8 in, 2 out]
  n110 = global write "RefNums_Sensors.vi" "Front-Right Prox Sensor"(w53) -> ()
  n111 = call <vilib>:"WPI_AnalogChannelRefNum Registry Set.vi"("refnum name"=w50, "AIDeviceRef"=w52) -> ()  [unwired: 8 in, 2 out]
  n112 = global write "RefNums_Sensors.vi" "Front-Left Prox Sensor"(w50) -> ()
  n113 = call <vilib>:"WPI_AnalogChannelRefNum Registry Set.vi"("refnum name"=w47, "AIDeviceRef"=w49) -> ()  [unwired: 8 in, 2 out]
  n114 = global write "RefNums_Sensors.vi" "Lower Pressure Transducer"(w47) -> ()
  n115 = call <vilib>:"WPI_AnalogChannelRefNum Registry Set.vi"("refnum name"=w44, "AIDeviceRef"=w46) -> ()  [unwired: 8 in, 2 out]
  n116 = global write "RefNums_Sensors.vi" "Lower Pressure Transducer"(w44) -> ()
  n117 = call <vilib>:"WPI_AnalogChannelRefNum Registry Set.vi"("refnum name"=w94, "AIDeviceRef"=w96) -> ()  [unwired: 8 in, 2 out]
  n118 = global write "RefNums_Sensors.vi" "Rear Prox Sensor"(w94) -> ()
  n119 = call <vilib>:"WPI_AnalogChannelRefNum Registry Set.vi"("refnum name"=w91, "AIDeviceRef"=w93) -> ()  [unwired: 8 in, 2 out]
  n120 = global write "RefNums_Sensors.vi" "Upper Pressure Transducer"(w91) -> ()
  n121 = global write "RefNums_Sensors.vi" "Left Prox Sensor"(w97) -> ()
  n122 = call <vilib>:"WPI_AnalogChannelRefNum Registry Set.vi"("refnum name"=w100, "AIDeviceRef"=w102) -> ()  [unwired: 8 in, 2 out]
  n123 = call <vilib>:"WPI_AnalogChannelRefNum Registry Set.vi"("refnum name"=w97, "AIDeviceRef"=w99) -> ()  [unwired: 8 in, 2 out]
  "error out" <- "error in"
